vi "Variant VI Tree.vi"   [LabVIEW 2016]
types:
  T1 = typedef "PSVARIANT_Data Type.ctl" = u8
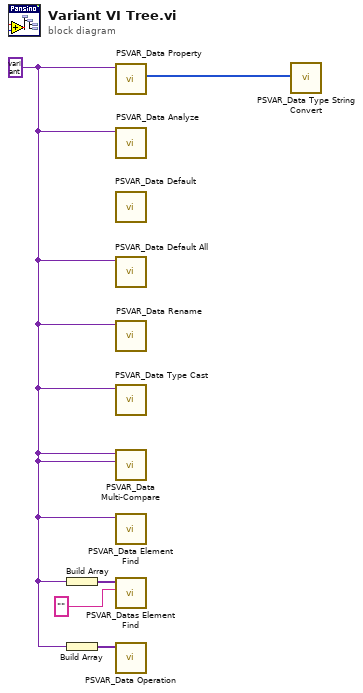
[diagram p0: block diagram]
diagram:
  w3 = variant ("Data")
  n1 = Build Array(w3) -> (w4:variant[])
  n2 = Build Array(w3) -> (w2:variant[])
  n3 = call "PSVAR_Data Property.vi"("Data"=w3) -> ("Type Data"=w5:T1[])  [unwired: 6 in, 4 out]
  n4 = call "PSVAR_Data Analyze.vi"("Data"=w3) -> ()  [unwired: 9 in, 2 out]
  n5 = call "PSVAR_Data Default.vi"() -> ()  [unwired: 10 in, 2 out]
  n6 = call "PSVAR_Data Default All.vi"("Data"=w3) -> ()  [unwired: 9 in, 2 out]
  n7 = call "PSVAR_Data Rename.vi"("Data In"=w3) -> ()  [unwired: 9 in, 2 out]
  n8 = call "PSVAR_Data Type Cast.vi"("Data In"=w3) -> ()  [unwired: 9 in, 2 out]
  n9 = call "PSVAR_Data Multi-Compare.vi"("Y"=w3, "X"=w3) -> ()  [unwired: 8 in, 2 out]
  n10 = call "PSVAR_Data Element Find.vi"("Data"=w3) -> ()  [unwired: 7 in, 4 out]
  n11 = call "PSVAR_Datas Element Find.vi"("Label"="", "Datas"=w4) -> ()  [unwired: 5 in, 5 out]
  n12 = call "PSVAR_Data Operation.vi"("Data In"=w2) -> ()  [unwired: 9 in, 2 out]
  n13 = call "PSVAR_Data Type String Convert.vi"("Type Array In"=w5) -> ()  [unwired: 8 in, 3 out]
